vi "03 - Intro to Events.vi"() -> ()   [LabVIEW 2019]
uses:
  Libraries/LibSDL2 Wrapper/Controls/Keyboard Event.ctl
  Libraries/LibSDL2 Wrapper/Controls/Mouse Motion Event.ctl
  Libraries/LibSDL2 Wrapper/Controls/Mouse Button Event.ctl
  Libraries/LibSDL2 Wrapper/Controls/Init Flags.ctl
  Libraries/LibSDL2 Wrapper/Controls/NULL.ctl
  Libraries/LibSDL2 Wrapper/LibSDL2.lvlib
panel:
  out "x-y":dbl
  out "Event Type":u32 format="%.0x"
  out "Mouse Button Event":T1
  out "Mouse Motion Event":T2
  out "Keyboard Event":T3 {"Padding 2" format="%.0x"; "Padding 1" format="%.0x"; "Window ID" format="%.0x"; "Type" format="%.0x"; "Key Sym"."Unused" format="%.0x"; "Key Sym"."Mod" format="%.0x"; "Key Sym"."Sym" format="%.0x"; "Key Sym"."Scan Code" format="%.0x"}
  out "Error":string
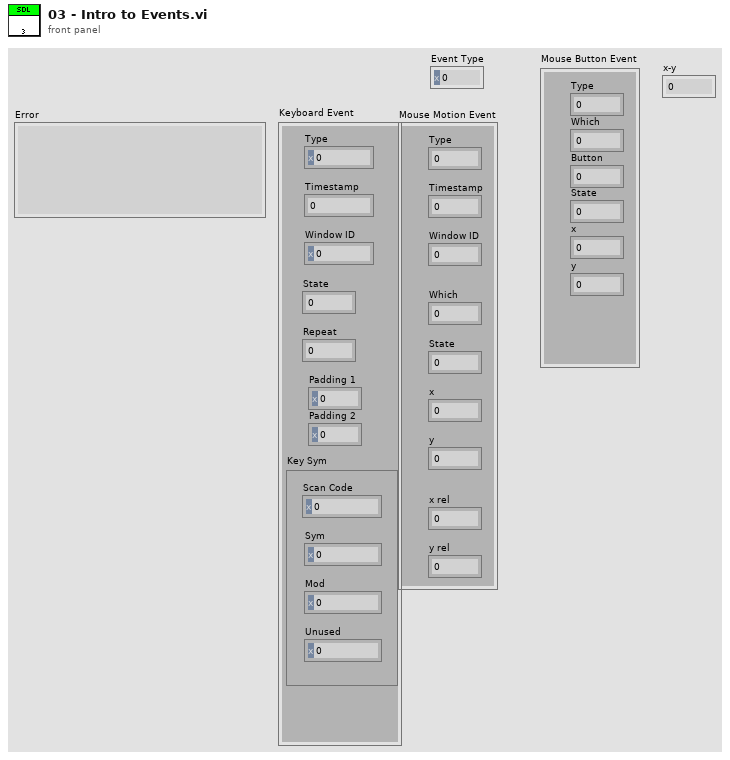
[diagram p1: front panel]
types:
  T1 = typedef "LibSDL2.lvlib/Mouse Button Event.ctl" = cluster{"Type":u8, "Which":u8, "Button":u8, "State":u8, "x":u16, "y":u16}
  T2 = typedef "LibSDL2.lvlib/Mouse Motion Event.ctl" = cluster{"Type":u32, "Timestamp":u32, "Window ID":u32, "Which":u32, "State":u32, "x":i32, "y":i32, "x rel":i32, "y rel":i32}
  T3 = typedef "LibSDL2.lvlib/Keyboard Event.ctl" = cluster{"Type":u32, "Timestamp":u32, "Window ID":u32, "State":u8, "Repeat":u8, "Padding 1":u8, "Padding 2":u8, "Key Sym":cluster{"Scan Code":u32, "Sym":i32, "Mod":u16, "Unused":u32}}
  T4 = typedef "LibSDL2.lvlib/Init Flags.ctl" = u32
  T5 = typedef "LibSDL2.lvlib/NULL.ctl" = enum32{"NULL"}
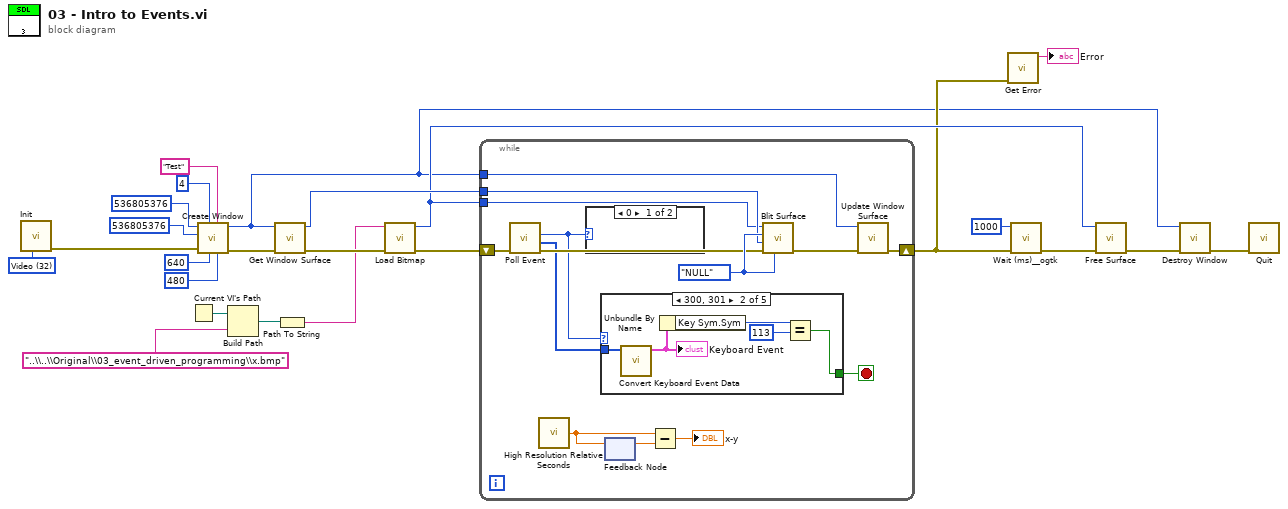
[diagram p0: block diagram]
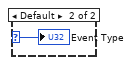
[diagram p2: hidden frame]
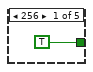
[diagram p3: hidden frame]
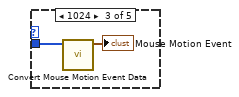
[diagram p4: hidden frame]
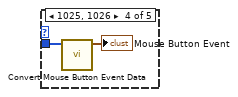
[diagram p5: hidden frame]
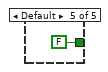
[diagram p6: hidden frame]
diagram:
  w24 = T4 32 items=["Timer"=1, "Audio"=16, "Video"=32, "Joystick"=512, "Haptic"=4096, "Game Controller"=8192, "Events"=16384, "No Parachute"=1048576, "Everything"=17244689] ("Init Flags")
  n1 = call "Init.vi"("Flags"=w24) -> ("error out"=w18:errorcluster)  [unwired: 9 in, 1 out]
  n2 = Current VI's Path() -> (path=w3:path)
  n3 = call "Create Window.vi"("Height"=480, "Title"="Test", "Width"=640, "Flags"=u32 4, "error in"=w18, "Position y"=u32 536805376 ("Flags"), "Position x"=u32 536805376 ("Flags")) -> ("error out"=w13:errorcluster, "Window Pointer"=w5:u32)  [unwired: 3 in]
  n4 = Build Path(base path=w3, name or relative path="..\\..\\Original\\03_event_driven_programming\\x.bmp" ("File")) -> (appended path=w4:path)
  n5 = call "Get Window Surface.vi"("error in"=w13, "Window Pointer"=w5) -> ("error out"=w12:errorcluster, "Surface Pointer"=w8:u32)  [unwired: 8 in]
  n6 = Path To String(path=w4) -> (string=w2:string)
  n7 = call "Load Bitmap.vi"("error in"=w12, "File"=w2) -> ("error out"=w11:errorcluster, "Surface Pointer"=w7:u32)  [unwired: 8 in]
  n8 = while {
    tunnel: w5 -> [w38]
    tunnel: w8 -> [w35]
    tunnel: w7 -> [w34]
    shift-right: [w33] -> w6
    shift-left: w11 -> [w32]
    stop <- w29 stop-if-true
    w36 = NULL."NULL" ("Null")
    n9 = call "Poll Event.vi"("error in"=w32) -> ("error out"=w31:errorcluster, "Event Data"=w30:u8[], "Event Type"=w28:u32)  [unwired: 7 in, 1 out]
    n10 = call <vilib>:"High Resolution Relative Seconds.vi"() -> ("relative seconds"=w27:dbl)
    n11 = case shown="0" w28 {
      selector: w28 -> [_ w39]
      frame 0 {
      }
      frame Default {
        "Event Type" <- w39
      }
    }
    n12 = case shown="300, 301" w28 {
      tunnel: w30 -> [_ w45 w47 w49 _]
      tunnel: [TRUE w41 _ _ FALSE] -> w29
      frame 256 {
      }
      frame 768, 769 {
        n13 = call "Convert Keyboard Event Data.vi"("Event Data"=w45) -> ("Keyboard Event"=w44:T3)  [unwired: 10 in]
        "Keyboard Event" <- w44
        n14 = Unbundle By Name(w44) -> ("Key Sym.Sym"=w43:i32)
        n15 = Equal?(x=w43, y=113) -> (x = y?=w41:bool)
      }
      frame 1024 {
        n16 = call "Convert Mouse Motion Event Data.vi"("Event Data"=w47) -> ("Mouse Motion Event"=→"Mouse Motion Event":T2)  [unwired: 10 in]
      }
      frame 1025, 1026 {
        n17 = call "Convert Mouse Button Event Data.vi"("Event Data"=w49) -> ("Mouse Button Event"=→"Mouse Button Event":T1)  [unwired: 10 in]
      }
      frame Default {
      }
    }
    n18 = feedback-in #1(w27) -> ()
    n19 = feedback #1() -> (w26:dbl)  [unwired: 1 in]
    n20 = Subtract(x=w27, y=w26) -> (x-y=→"x-y":dbl)
    n21 = call "Blit Surface.vi"("Destination Rectangle Pointer"=w36, "error in"=w31, "Destination Surface Pointer"=w35, "Source Rectangle Pointer"=w36, "Source Surface Pointer"=w34) -> ("error out"=w37:errorcluster)  [unwired: 5 in, 1 out]
    n22 = call "Update Window Surface.vi"("error in"=w37, "Window Pointer"=w38) -> ("error out"=w33:errorcluster)  [unwired: 9 in]
  }
  n23 = call "Get Error.vi"("error in"=w6) -> ("Error"=→"Error":string)  [unwired: 9 in, 1 out]
  n24 = call <userlib>:"Wait (ms)__ogtk.vi"("error in (no error)"=w6, "milliseconds to wait"=u32 1000) -> ("error out"=w10:errorcluster)  [unwired: 8 in, 1 out]
  n25 = call "Free Surface.vi"("error in"=w10, "Surface Pointer"=w7) -> ("error out"=w9:errorcluster)  [unwired: 9 in]
  n26 = call "Destroy Window.vi"("error in"=w9, "Window Pointer"=w5) -> ("error out"=w15:errorcluster)  [unwired: 9 in]
  n27 = call "Quit.vi"("error in"=w15) -> ()  [unwired: 10 in, 1 out]
